vi "Write Exposure Time abs Attr.vi"(8 "error in (no error)":errorcluster, 10 "Exposure Time abs Attr":string="CameraAttributes::AcquisitionTrigger::ExposureTimeAbs", 11 "Camera Quick Settings Panel in":refnum<class "Camera Quick Settings Panel.lvclass">) -> (0 "error out":errorcluster, 3 "Camera Quick Settings Panel out":refnum<class "Camera Quick Settings Panel.lvclass">)   [LabVIEW 2014, in "Camera Quick Settings Panel.lvlib" / "Camera Quick Settings Panel.lvclass"]
uses:
  Camera Quick Settings Panel.lvclass
  Camera Quick Settings Panel.lvclass/Camera Quick Settings Panel.ctl
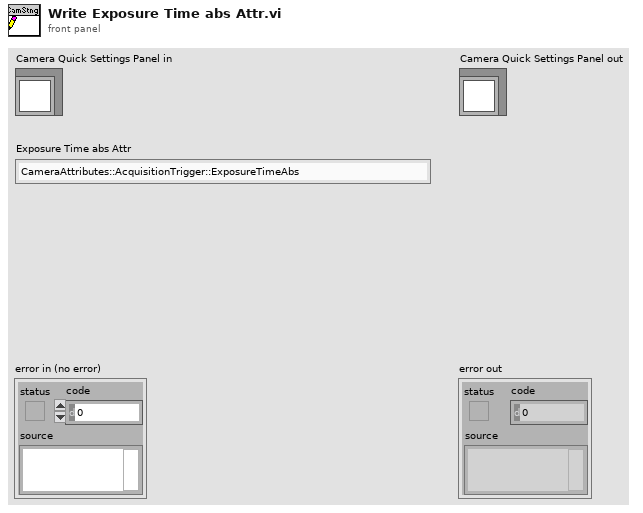
[diagram p1: front panel]
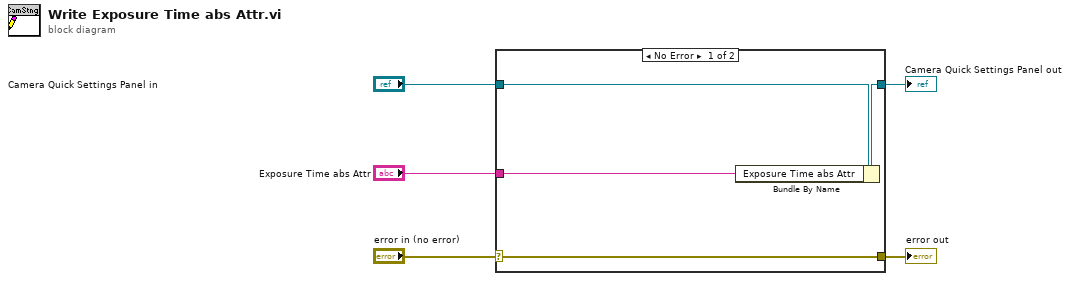
[diagram p0: block diagram]
diagram:
  n1 = case shown="No Error" "error in (no error)" {
    selector: "error in (no error)" -> [w9 w10]
    tunnel: [w9 w10] -> w4
    tunnel: [w7 w11] -> w2
    tunnel: "Camera Quick Settings Panel in" -> [w8 w11]
    tunnel: "Exposure Time abs Attr" -> [w6 _]
    frame No Error {
      n2 = Bundle By Name(cluster=w8, "Exposure Time abs Attr"=w6) -> (w7:refnum<class "Camera Quick Settings Panel.lvclass">)
    }
    frame Error {
    }
  }
  "error out" <- w4
  "Camera Quick Settings Panel out" <- w2
